vi "Get Items from File.vi"(8 "Error in":errorcluster) -> (0 "Error out":errorcluster, 3 "Items":T1(array[cluster]) {"Data type" items=["Boolean"=1, "SByte"=2, "Byte"=3, "Int16"=4, "UInt16"=5, "Int32"=6, "UInt32"=7, "Int64"=8, "UInt64"=9, "Float"=10, "Double"=11, "String"=12, "DateTime"=13, "ByteString"=15, "Array of Boolean"=101, "Array of SByte"=102, "Array of Byte"=103, "Array of Int16"=104, "Array of UInt16"=105, "Array of Int32"=106, "Array of UInt32"=107, "Array of Int64"=108, "Array of UInt64"=109, "Array of Float"=110, "Array of Double"=111, "Array of String"=112, "Array of DateTime"=113, "Array of ByteString"=115]; "Access level" items=["read-only"=1, "write-only"=2, "read/write"=3]})   [LabVIEW 2020]
uses:
  <vilib>/Utility/config.llb/Read Key (String).vi
  <vilib>/Utility/config.llb/NI_LVConfig.lvlib
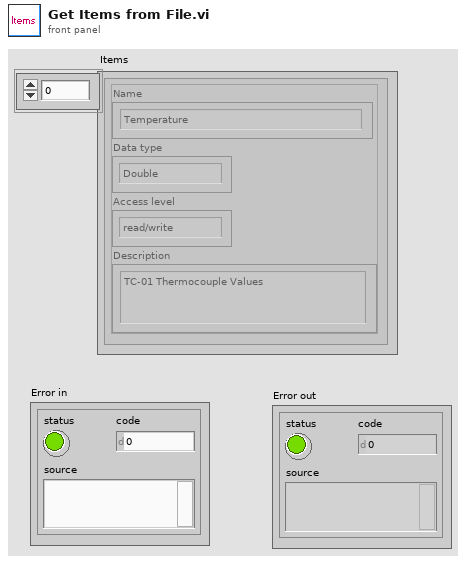
[diagram p1: front panel]
types:
  T1 = cluster{"Name":string, "Data type":u16, "Access level":u16, "Description":string}[]
  T2 = typedef "NI_LVConfig.lvlib/Config Data RefNum.ctl" = refnum<k1>
  T3 = cluster{"Name":string, "Data type":u16, "Access level":u16, "Description":string}
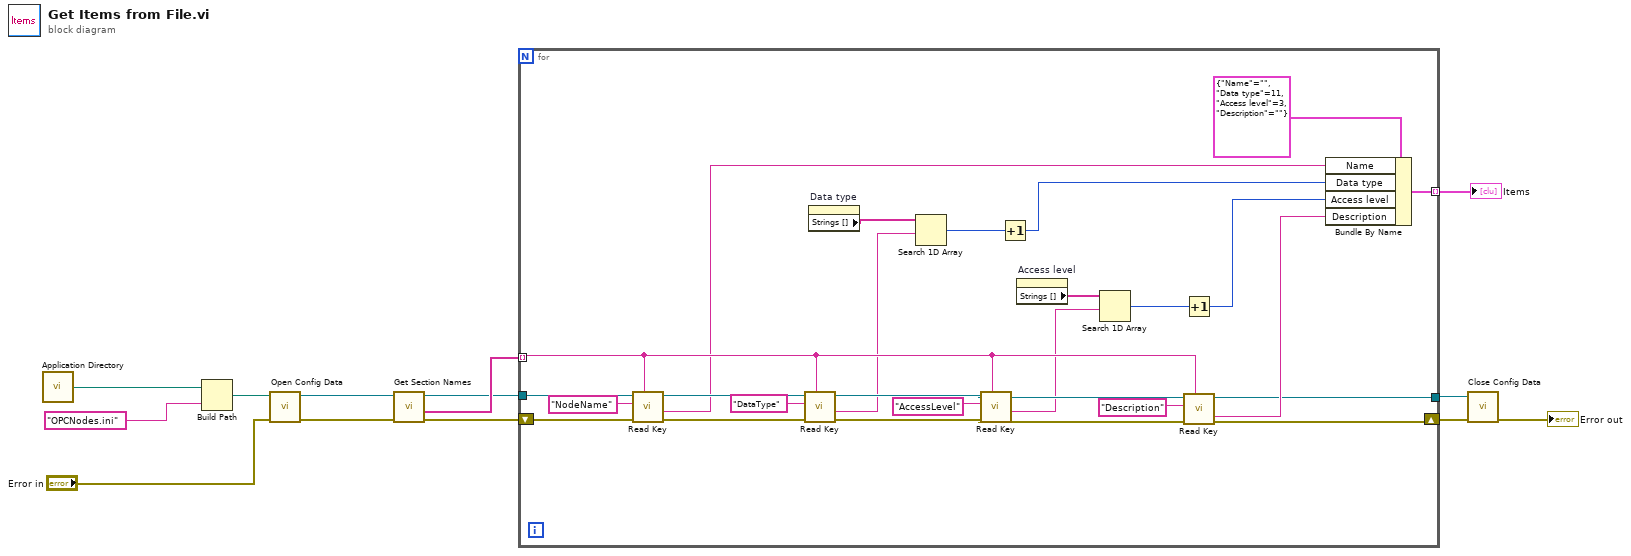
[diagram p0: block diagram]
diagram:
  n1 = call <vilib>:"Application Directory.vi"() -> ("Application Directory"=w13:path)
  n2 = Build Path(base path=w13, name or relative path="OPCNodes.ini") -> (appended path=w11:path)
  n3 = call <vilib>:"Open Config Data.vi"("error in (no error)"="Error in", "configuration file path"=w11) -> ("error out"=w10:errorcluster, "refnum"=w7:T2)  [unwired: 7 in, 1 out]
  n4 = call <vilib>:"Get Section Names.vi"("error in (no error)"=w10, "refnum"=w7) -> ("error out"=w9:errorcluster, "section names"=w6:string[], "refnum out"=w5:T2)  [unwired: 7 in]
  n5 = for {
    shift-right: [w25] -> w8
    shift-left: w9 -> [w40]
    tunnel: w6 -> [w31] mode=indexing
    tunnel: w5 -> [w39]
    tunnel: [w24] -> w4
    tunnel: [w16] -> w3 mode=indexing
    n6 = call-poly <vilib>:"Read Key.vi"("section"=w31, "error in (no error)"=w40, "key"="NodeName", "refnum"=w39) -> ("error out"=w30:errorcluster, "value"=w27:string, "refnum out"=w34:T2)  [unwired: 4 in, 1 out]
    n7 = call-poly <vilib>:"Read Key.vi"("section"=w31, "error in (no error)"=w30, "key"="DataType", "refnum"=w34) -> ("error out"=w29:errorcluster, "value"=w22:string, "refnum out"=w33:T2)  [unwired: 4 in, 1 out]
    n8 = property on="Data type" class="Ring (strict)"() -> ("Strings []"=w14:string[])  [unwired: 2 in, 2 out]
    n9 = Search 1D Array(1D array=w14, element=w22) -> (index of element=w23:i32)  [unwired: 1 in]
    n10 = call-poly <vilib>:"Read Key.vi"("section"=w31, "error in (no error)"=w29, "key"="AccessLevel", "refnum"=w33) -> ("error out"=w28:errorcluster, "value"=w18:string, "refnum out"=w32:T2)  [unwired: 4 in, 1 out]
    n11 = Increment(x=w23) -> (x+1=w19:i32)
    n12 = property on="Access level" class="Ring (strict)"() -> ("Strings []"=w20:string[])  [unwired: 2 in, 2 out]
    n13 = Search 1D Array(1D array=w20, element=w18) -> (index of element=w21:i32)  [unwired: 1 in]
    n14 = Increment(x=w21) -> (x+1=w17:i32)
    n15 = call-poly <vilib>:"Read Key.vi"("section"=w31, "error in (no error)"=w28, "key"="Description", "refnum"=w32) -> ("error out"=w25:errorcluster, "value"=w26:string, "refnum out"=w24:T2)  [unwired: 4 in, 1 out]
    n16 = Bundle By Name(cluster=T3 {"Name"="", "Data type"=11, "Access level"=3, "Description"=""} ("Item 2"), "Name"=w27, "Data type"=w19, "Access level"=w17, "Description"=w26) -> (w16:T3)
  }
  "Items" <- w3
  n17 = call <vilib>:"Close Config Data.vi"("error in (no error)"=w8, "refnum"=w4) -> ("error out"=→"Error out":errorcluster)  [unwired: 8 in, 1 out]
